vi "ChamberTempTCPRead_v1.vi"() -> ()   [LabVIEW 2010]
panel:
  in  "file path (use dialog)":path
  out "output array":dbl[](array[numeric])
  out "Waveform Chart":dbl(graph)
  in  "address":string
  in  "bytes to read":i32
  in  "Disconnect":bool
  in  "Port":u16
  in  "length 2":i32
  in  "offset 2":i32
  out "Temp 2 DBL":dbl
  out "Temperature String 2":string
  in  "length 1":i32
  in  "offset 1":i32
  out "Temperature DBL":dbl
  out "Temperature String":string
  in  "Mode (standard)":T1(ring)
  out "Data In":string
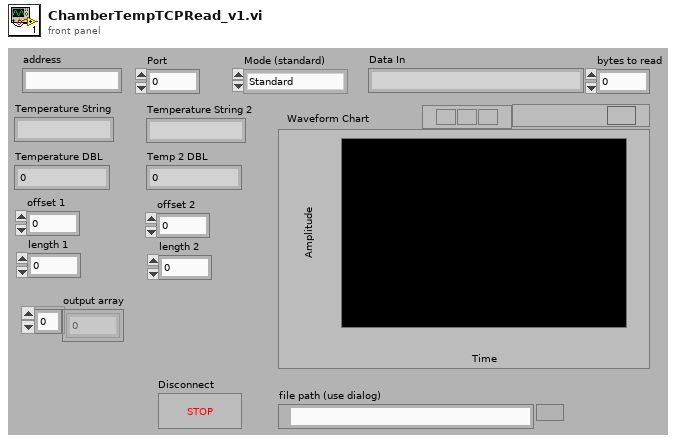
[diagram p1: front panel]
types:
  T1 = enum16{"Standard", "Buffered", "CRLF", "Immediate"}
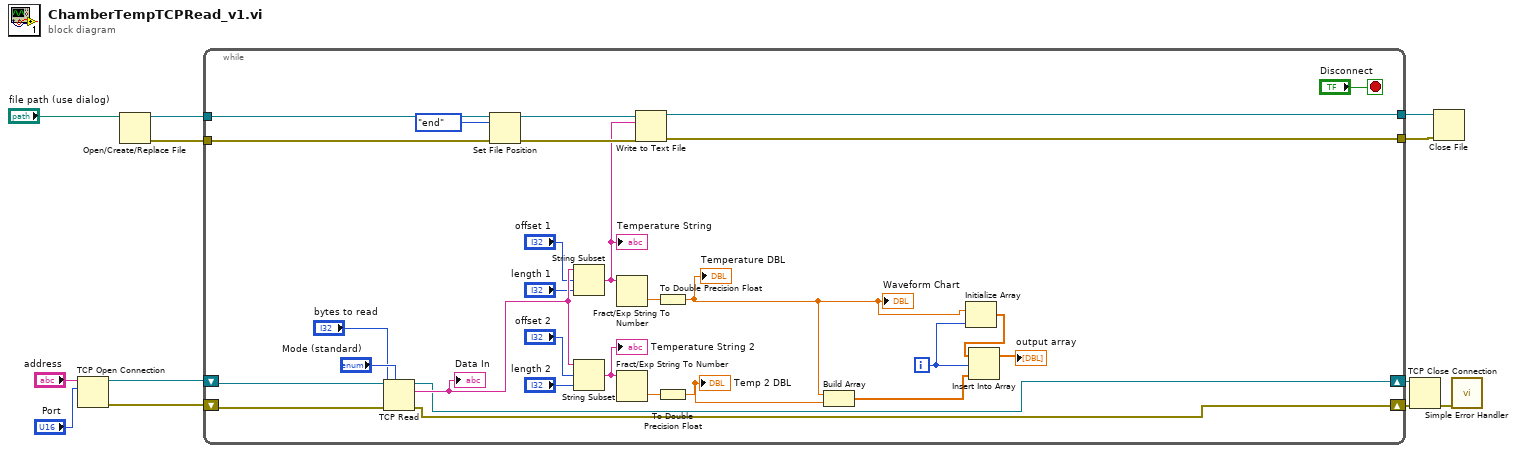
[diagram p0: block diagram]
diagram:
  n1 = TCP Open Connection(address="address", remote port or service name="Port") -> (connection ID=w11:refnum<k5>, error out=w10:errorcluster)  [unwired: 3 in]
  n2 = Open/Create/Replace File(file path (use dialog)="file path (use dialog)") -> (refnum out=w5:refnum<file>, error out=w4:errorcluster)  [unwired: 5 in, 1 out]
  n3 = while {
    shift-right: [w26] -> w8
    shift-left: w11 -> [w41]
    shift-right: [w25] -> w6
    shift-left: w10 -> [w40]
    tunnel: w5 -> [w16]
    tunnel: w4 -> [w15]
    tunnel: [w14] -> w3
    tunnel: [w13] -> w2
    i -> [w23]
    stop <- "Disconnect" stop-if-true
    n4 = TCP Read(connection ID=w41, bytes to read="bytes to read", error in (no error)=w40, 7:"Mode (standard)") -> (connection ID out=w26:refnum<k5>, data out=w39:string, error out=w25:errorcluster)  [unwired: 1 out]
    "Data In" <- w39
    n5 = Set File Position(refnum=w16, from (0:start)=enum16{"start", "end", "current"}."end", error in=w15) -> (refnum out=w24:refnum<file>, error out=w27:errorcluster)  [unwired: 1 in]
    n6 = String Subset(string=w39, offset (0)="offset 1", length (rest)="length 1") -> (substring=w18:string)
    "Temperature String" <- w18
    n7 = String Subset(string=w39, offset (0)="offset 2", length (rest)="length 2") -> (substring=w29:string)
    "Temperature String 2" <- w29
    n8 = Fract/Exp String To Number(string=w18) -> (number=w32:dbl)  [unwired: 3 in, 1 out]
    n9 = Fract/Exp String To Number(string=w29) -> (number=w35:dbl)  [unwired: 3 in, 1 out]
    n10 = Write to Text File(file (use dialog)=w24, text=w18, error in=w27) -> (refnum out=w13:refnum<file>, error out=w14:errorcluster)  [unwired: 1 in, 1 out]
    n11 = To Double Precision Float(number=w32) -> (double precision float=w19:dbl)
    "Temperature DBL" <- w19
    "Waveform Chart" <- w19
    n12 = To Double Precision Float(number=w35) -> (double precision float=w21:dbl)
    "Temp 2 DBL" <- w21
    n13 = Build Array "Build Array"(w19, w21) -> (w22:dbl[])
    n14 = Initialize Array(w19, w23) -> (w20:dbl[])
    n15 = Insert Into Array(array=w20, index=w23, new element=w22) -> (→"output array":dbl[])
  }
  n16 = TCP Close Connection(connection ID=w8, error in (no error)=w6) -> (error out=w12:errorcluster)  [unwired: 2 out]
  n17 = Close File(refnum=w2, error in=w3) -> ()  [unwired: 2 out]
  n18 = call <vilib>:"Simple Error Handler.vi"("error in (no error)"=w12) -> ()  [unwired: 1 in, 8 out]
